vi "Create.vi"(8 "error in (no error)":errorcluster) -> (0 "error out":errorcluster, 3 "Single Thread Test Runner out":refnum<class "Single Thread Test Runner.lvclass">)   [LabVIEW 2020, in "Single Thread Test Runner.lvclass"]
uses:
  Single Thread Test Runner.lvclass
  Single Thread Test Runner.lvclass/Single Thread Test Runner.ctl
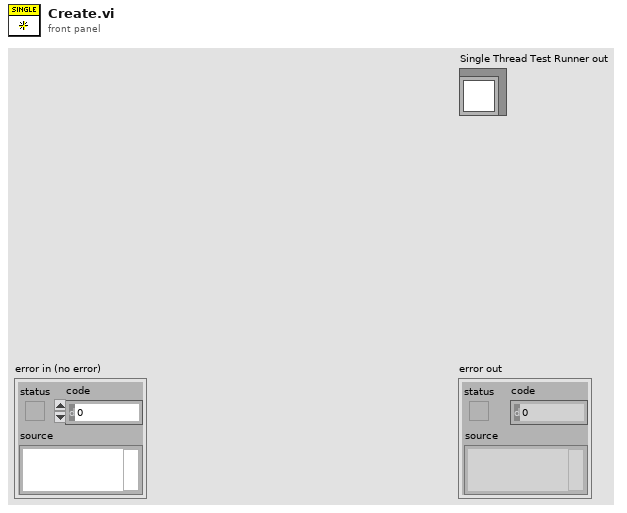
[diagram p1: front panel]
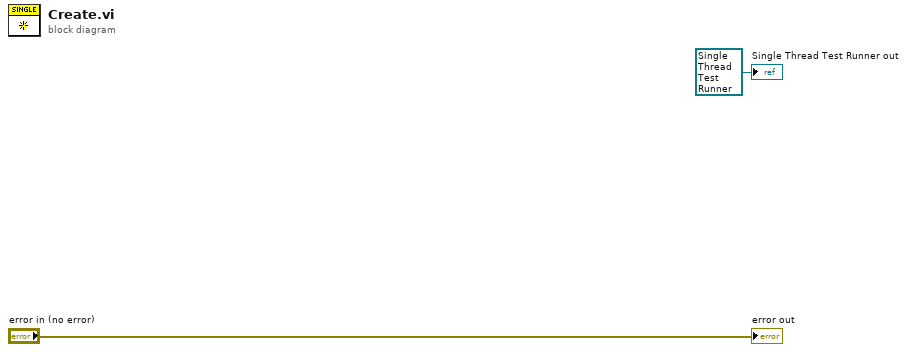
[diagram p0: block diagram]
diagram:
  "error out" <- "error in (no error)"
  "Single Thread Test Runner out" <- refnum<class "Single Thread Test Runner.lvclass"> refnum ("Single Thread Test Runner out")
